vi "M_alpha_beta (SubVI).vi"(4 "i":i32, 6 "Sref":dbl, 7 "FE [N]":dbl[](array[numeric]), 9 "le [m]":dbl, 10 "Data":dbl[][](array[numeric]), 11 "Pdin [Pa]":dbl) -> (2 "M_beta":dbl, 3 "M_alpha":dbl)   [LabVIEW 2017]
uses:
  <vilib>/Analysis/_algsub.llb/Vector Norm Type.ctl
  <vilib>/Analysis/_algsub.llb/Real Vector Norm.vi
  <vilib>/Analysis/NI_AALPro.lvlib
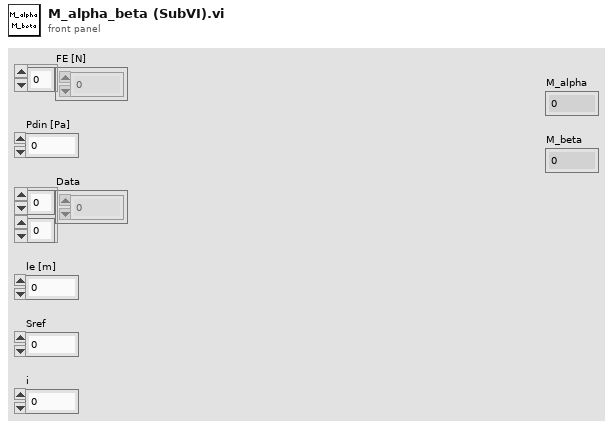
[diagram p1: front panel]
types:
  T1 = typedef "NI_AALPro.lvlib/Vector Norm Type.ctl" = u16
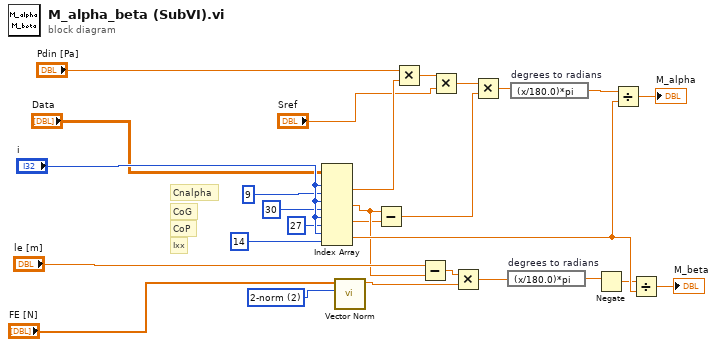
[diagram p0: block diagram]
diagram:
  w18 = T1 2 items=["1-norm"=1, "2-norm"=2, "Inf-norm"=3, "-Inf-norm"=4, "User Defined"=5] ("norm type")
  # "Ixx"
  # "CoP"
  # "CoG"
  # "Cnalpha"
  n1 = Index Array(array="Data", index (row) #1="i", index (col) #1=9 ("disabled index (col)"), index (row) #2="i", index (col) #2=30 ("disabled index (col)"), index (row) #3="i", index (col) #3=27 ("disabled index (col)"), index (row) #4="i", index (col) #4=14 ("disabled index (col)")) -> (element #1=w15:dbl, element #2=w19:dbl, element #3=w10:dbl, element #4=w26:dbl)
  n2 = call-poly <vilib>:"Vector Norm.vi"("norm type"=w18, "Input Vector"="FE [N]") -> ("norm"=w20:dbl)  [unwired: 8 in, 1 out]
  n3 = Subtract(x=w19, y=w10) -> (x-y=w12:dbl)
  n4 = Multiply(x="Pdin [Pa]", y=w15) -> (x*y=w8:dbl)
  n5 = Subtract(x="le [m]", y=w19) -> (x-y=w21:dbl)
  n6 = Multiply(x=w8, y="Sref") -> (x*y=w11:dbl)
  n7 = Multiply(x=w21, y=w20) -> (x*y=w23:dbl)
  n8 = Multiply(x=w11, y=w12) -> (x*y=w13:dbl)
  n9 = expression code="(x/180.0)*pi" "degrees to radians"(w23) -> (w24:dbl)
  n10 = expression code="(x/180.0)*pi" "degrees to radians"(w13) -> (w14:dbl)
  n11 = Negate(x=w24) -> (-x=w25:dbl)
  n12 = Divide(x=w14, y=w26) -> (x/y=→"M_alpha":dbl)
  n13 = Divide(x=w25, y=w26) -> (x/y=→"M_beta":dbl)
